vi "运维调试_CODCr.vi"() -> ()   [LabVIEW 2016, in "CODCr库.lvlib"]
uses:
  <vilib>/Utility/miscctls.llb/LVPointTypeDef.ctl
  <vilib>/ptbypt/NI_PtbyPt.lvlib
  <vilib>/Utility/config.llb/NI_LVConfig.lvlib
panel:
  in  "手动模式":bool
  in  "维护模式":bool
  out "数据时间":timestamp format="%<%Y/%m/%d %H:%M:%S>T"
  in  "质控参数":bool
  in  "仪器参数":bool
  in  "MB通信方式选择":enum16{"串口", "TCP"}(ring)
  in  "释放串口":bool
  in  "打开串口":bool
  in  "加标回收测试":bool
  in  "平行样测试":bool
  in  "定时启动":bool
  out "COM口":string
  in  "空白测试":bool
  in  "隐藏按钮":bool
  in  "写入消解温度时长":bool
  in  "保存KB值":bool
  in  "标样核查":bool
  out "启动时间":timestamp format="%<%Y/%m/%d %H:%M:%S>T"
  out "主循环次数":i32
  out "status":bool
  out "启动测量模式":T1(ring)
  out "曲线截距B":sgl format="%#_10g"
  out "曲线斜率K":sgl format="%#_10g"
  out "量程上限":sgl
  out "量程下限":sgl
  out "消解时长":u16
  out "消解温度":u16
  out "测量精度":u16
  out "测量结果":sgl
  out "标样参考值":sgl
  out "量程":u16
  out "工作状态":T1(ring)
  out "仪器时间":timestamp format="%<%X\n%x>T"
  out "关键参数区":T2
  out "状态告警区":T3 {"告警代码" items=["无告警", "缺试剂告警", "缺水样告警", "缺蒸馏水告警", "缺标液告警", "仪表漏液告警", "标定异常告警", "超量程告警", "加热异常", "低试剂预警", "超上限告警", "超下限告警", "仪表内部其他异常", "滴定异常告警", "电极异常告警", "量程切换告警", "参数设置告警", "PH电极电位异常", "电导率电极异常", "浊度光度异常", "溶解氧电极异常", "溶解氧光强异常", "温度异常告警", "PH异常告警", "溶解氧异常告警", "电导率异常告警", "浊度异常告警", "叶绿素异常告警", "藻密度异常告警", "蓝绿藻异常告警", "ORP异常告警", "氨氮异常告警", "清洁刷异常告警", "SD卡异常告警", "蓝牙异常告警", "Wifi异常告警", "流程异常告警"]; "故障代码" items=["无故障", "电机故障", "温度故障", "通讯故障", "滴定故障"]}
  out "测量数据区":T4 {"单位" items=["ug/L", "mg/L", "ppm", "mg/m3", "cm", "ppb", "ug/m3", "%", "nmol/mol", "umol/mol", "MPN/L", "MPN/100ml", "ng/m3", "NTU", "无量纲", "ms/cm", "us/cm", "℃", "mV", "万个/L"]}
  out "系统时间":timestamp format="%<%Y/%m/%d %H:%M:%S>T"
  in  "停止":bool
  in  "校时":bool
  in  "标样校准":bool
  in  "空白校准":bool
  in  "零点核查":bool
  in  "跨度核查":bool
  in  "水样测试":bool
  in  "返回":bool
  in  "设置":bool
  # "mg/L"
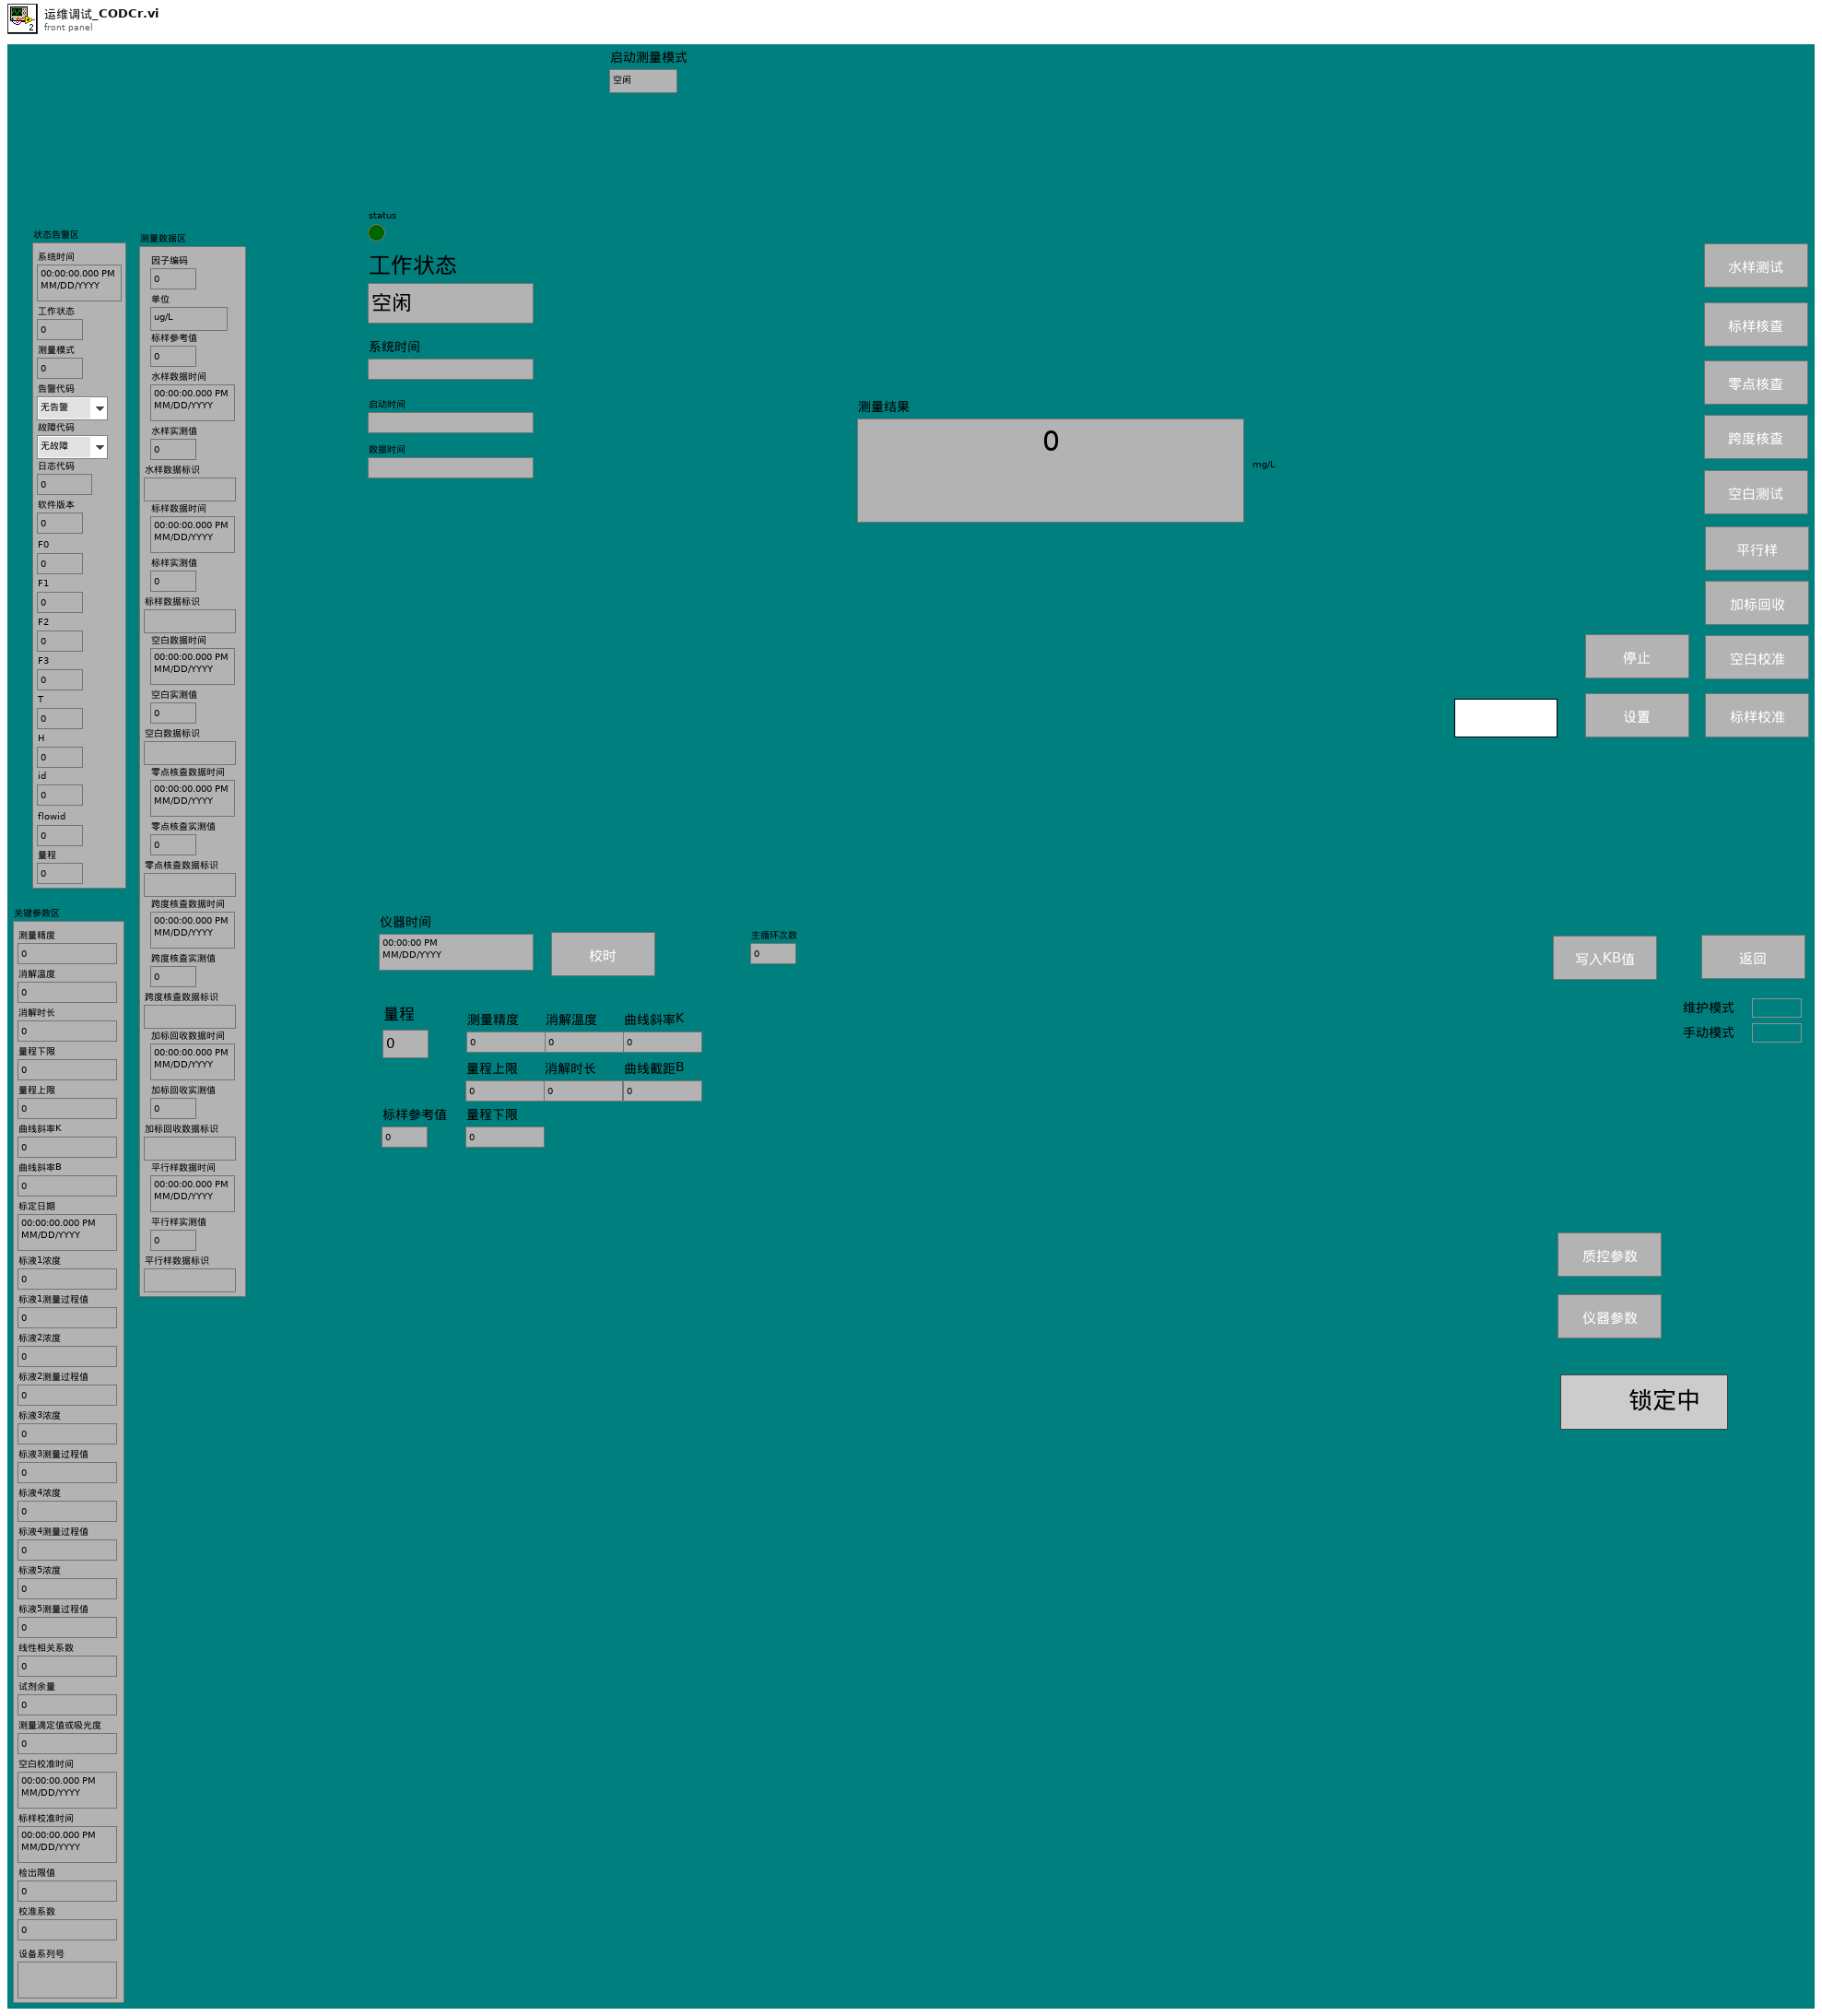
[diagram p1: front panel]
types:
  T1 = enum16{"空闲", "水样测试", "标样核查", "零点核查", "跨度核查", "空白测试", "平行样测试", "加标回收", "空白校准", "标样校准", "初始化（清洗）"}
  T2 = cluster{"测量精度":u16, "消解温度":u16, "消解时长":u16, "量程下限":sgl, "量程上限":sgl, "曲线斜率K":sgl, "曲线斜率B":sgl, "标定日期":timestamp, "标液1浓度":sgl, "标液1测量过程值":sgl, "标液2浓度":sgl, "标液2测量过程值":sgl, "标液3浓度":sgl, "标液3测量过程值":sgl, "标液4浓度":sgl, "标液4测量过程值":sgl, "标液5浓度":sgl, "标液5测量过程值":sgl, "线性相关系数":sgl, "试剂余量":u32, "测量滴定值或吸光度":sgl, "空白校准时间":timestamp, "标样校准时间":timestamp, "检出限值":sgl, "校准系数":sgl, "设备系列号":string}
  T3 = cluster{"系统时间":timestamp, "工作状态":u16, "测量模式":u16, "告警代码":u16, "故障代码":u16, "日志代码":u16, "软件版本":u16, "F0":sgl, "F1":sgl, "F2":sgl, "F3":sgl, "T":sgl, "H":sgl, "id":u16, "flowid":u16, "量程":u16}
  T4 = cluster{"因子编码":u32, "单位":u16, "标样参考值":sgl, "水样数据时间":timestamp, "水样实测值":sgl, "水样数据标识":string, "标样数据时间":timestamp, "标样实测值":sgl, "标样数据标识":string, "空白数据时间":timestamp, "空白实测值":sgl, "空白数据标识":string, "零点核查数据时间":timestamp, "零点核查实测值":sgl, "零点核查数据标识":string, "跨度核查数据时间":timestamp, "跨度核查实测值":sgl, "跨度核查数据标识":string, "加标回收数据时间":timestamp, "加标回收实测值":sgl, "加标回收数据标识":string, "平行样数据时间":timestamp, "平行样实测值":sgl, "平行样数据标识":string}
  T5 = cluster{"命令":string, "测量模式":enum16{"水样测量", "标样核查", "零点核查", "跨度核查", "空白测试", "加标回收", "平行样", "校零", "校标"}, "CODCr量程切换":enum32{"H", "L", "AUTO"}}
  T6 = typedef "LVPointTypeDef.ctl" = cluster{"Horizontal":i16, "Vertical":i16}
  T7 = typedef "NI_LVConfig.lvlib/Config Data RefNum.ctl" = refnum<k1>
  T8 = typedef "报警信息字段定义.ctl" = cluster{"时间":timestamp, "参数":string, "元器件":string, "故障现象":string, "故障分析":string, "state":string, "code":string, "platform_alarm_code":string}
  T9 = cluster{"时间标识":timestamp, "参数":string, "日志信息":string, "流程参数":string}
  T10 = cluster{"测量模式":enum16{"水样测量", "标样核查", "零点核查", "跨度核查", "空白测试", "加标回收", "平行样", "校零", "校标"}}
  T11 = typedef "TimingControl.lvlib/TimingControl.lvclass/国标控制命令.ctl" = enum16{"启动测量", "标样核查", "零点核查", "跨度核查", "空白测试", "平行样测试", "加标回收", "空白校准", "标样校准", "初始化（清洗）", "停止测试", "仪器重启", "校时", "模式设置", "测量间隔设置"}
  T12 = typedef "TimingControl.lvlib/TimingControl.lvclass/测量参数.ctl" = u16
  T13 = cluster{"测量量程":dbl, "测量精度":dbl, "测量间隔":dbl, "消解温度":dbl, "消解时长":dbl, "空白校准时间":timestamp, "曲线截距":dbl, "曲线斜率":dbl, "测量检出限":dbl, "测量信号值":dbl, "线性相关系数":dbl, "二次多项式系数":dbl, "标样校准时间":timestamp, "稀释倍数":dbl, "三项式系数":dbl, "空白标定系数":dbl, "量程系数":dbl}
  T14 = cluster{"确定":bool, "测量量程":dbl, "测量精度":dbl, "测量间隔":dbl, "消解温度":dbl, "消解时长":dbl, "空白校准时间":timestamp, "曲线截距":dbl, "曲线斜率":dbl, "测量检出限":dbl, "测量信号值":dbl, "线性相关系数":dbl, "二次多项式系数":dbl, "标样校准时间":timestamp, "稀释倍数":dbl, "三项式系数":dbl, "空白标定系数":dbl, "量程系数":dbl}
  T15 = cluster{"跨度值":dbl, "零点标准液浓度":dbl, "跨度标准液浓度":dbl, "标准液标准浓度":dbl}
  T16 = cluster{"确定":bool, "跨度值":dbl, "零点标准液浓度":dbl, "跨度标准液浓度":dbl, "标准液标准浓度":dbl}
  T17 = enum16{"水样测量", "标样核查", "零点核查", "跨度核查", "空白测试", "加标回收", "平行样", "校零", "校标"}
  T18 = typedef "CODCr库.lvlib/测试模式.ctl" = enum16{"N", "M"}
  T19 = cluster{"运行模式":enum16{"维护模式", "常规模式", "应急模式", "质控模式"}}
  T20 = cluster{"时间标识":timestamp, "监测值":sgl, "单位":u16, "数据标识":string, "因子编码":u32, "标样参考值":sgl, "F0":sgl, "F1":sgl, "F2":sgl, "F3":sgl, "温度":sgl, "湿度":sgl, "量程标识":string, "LastTime":timestamp}
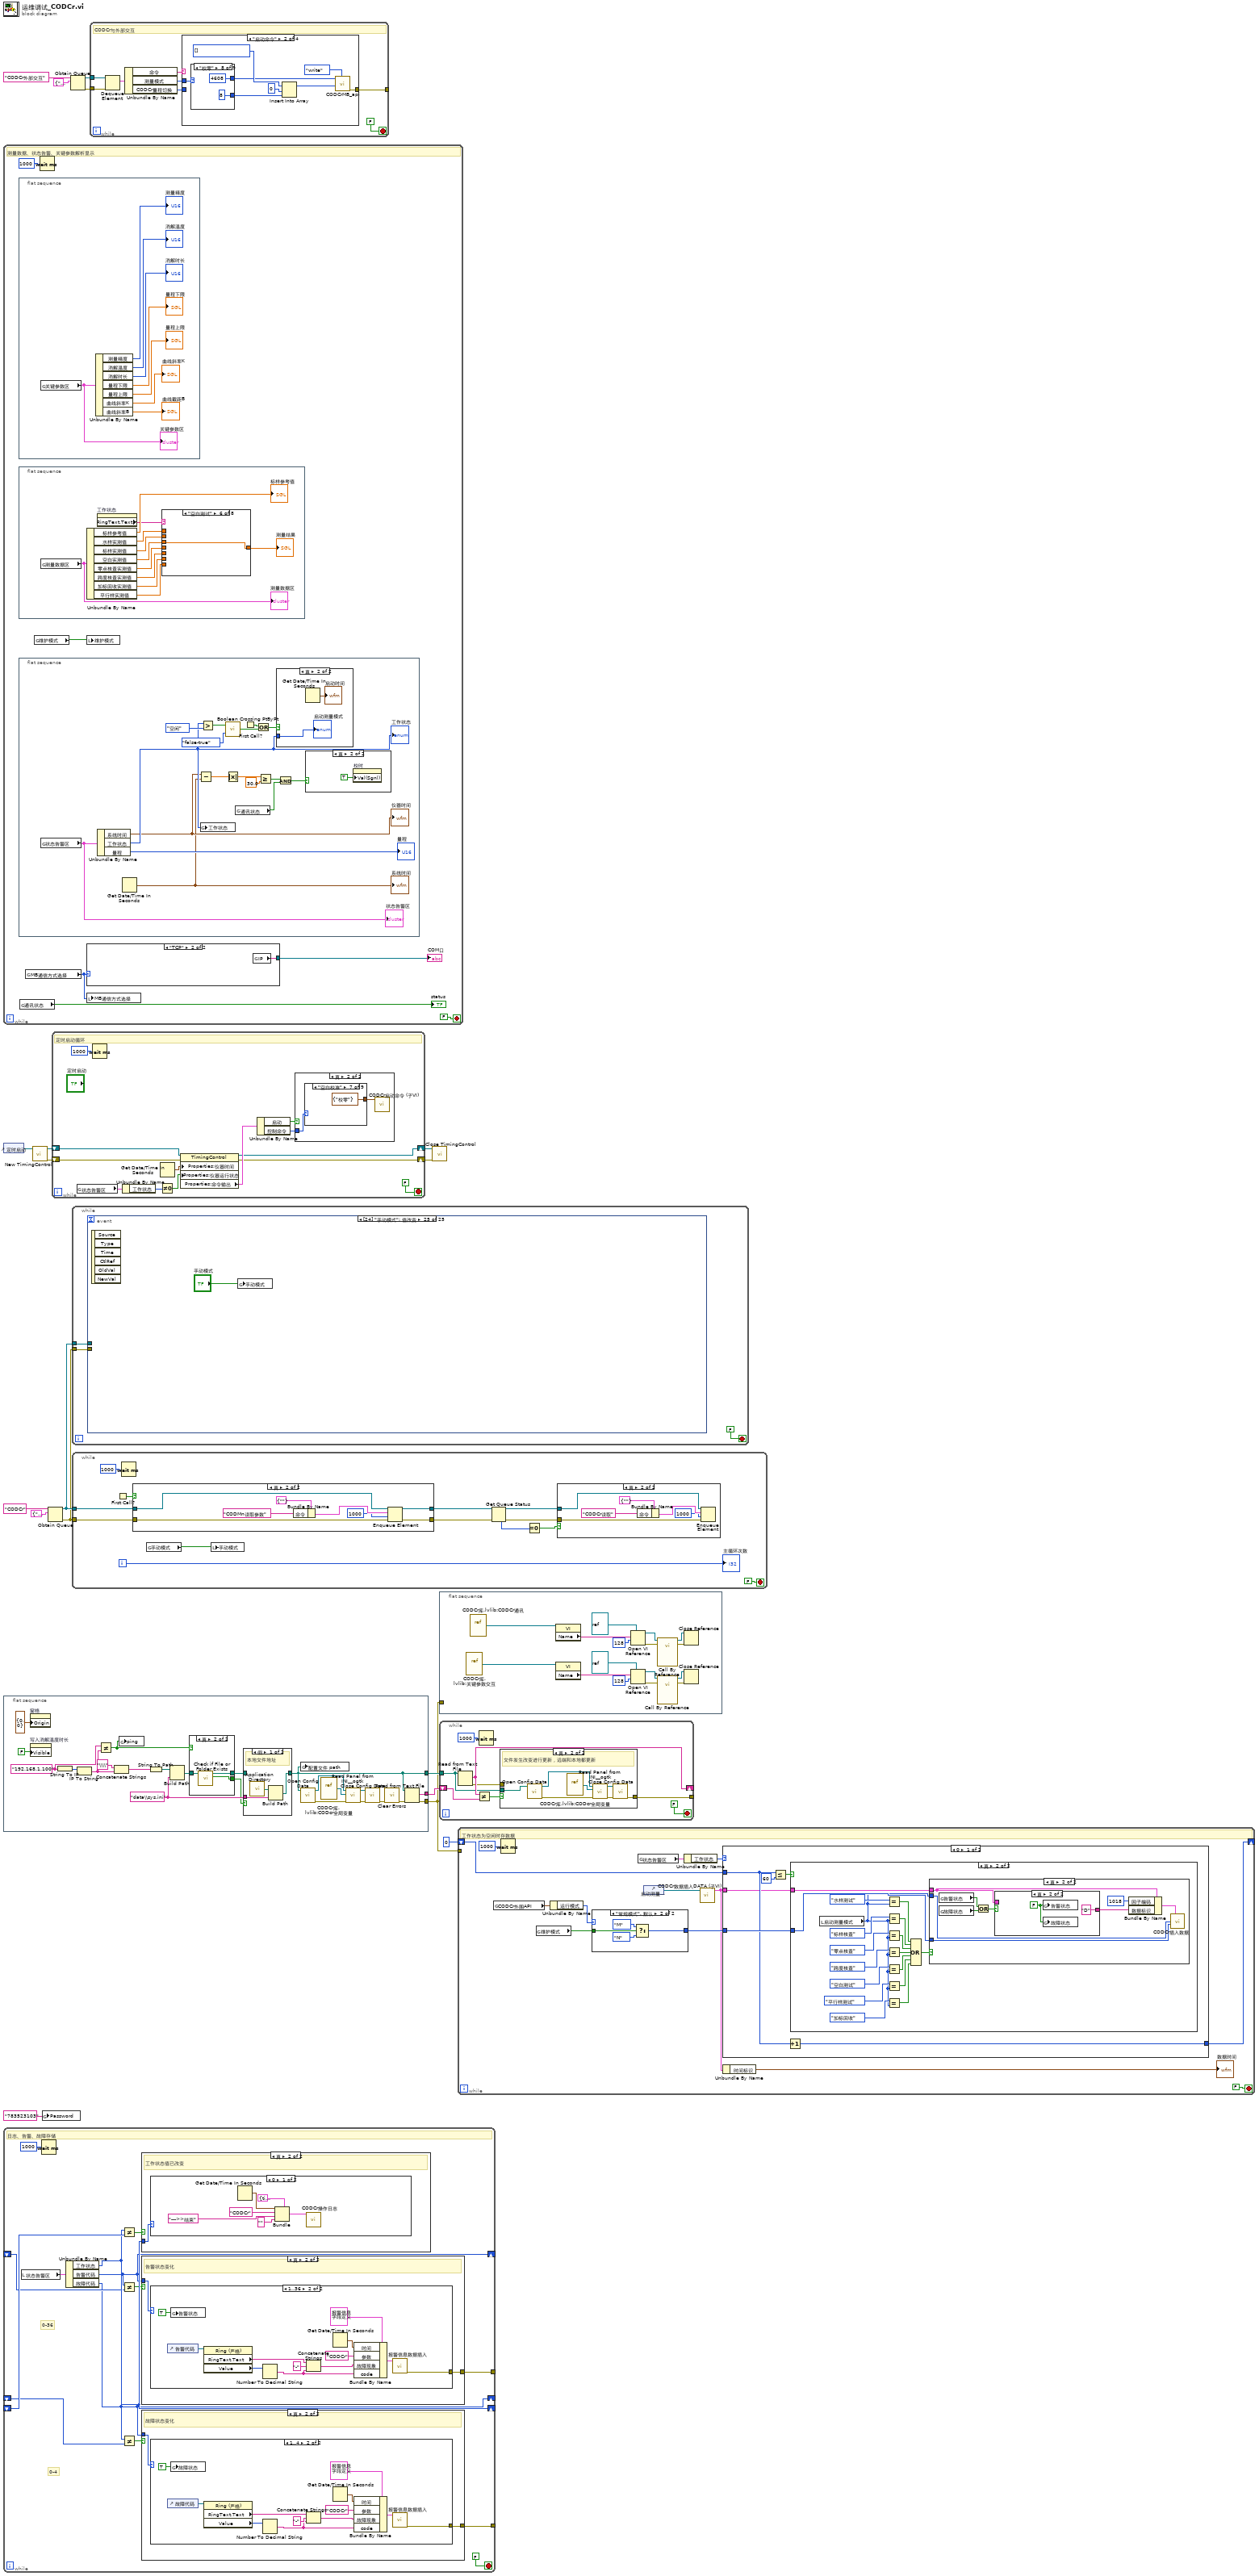
[diagram p0: block diagram]
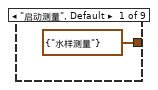
[diagram p3: hidden frame]
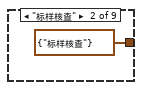
[diagram p4: hidden frame]
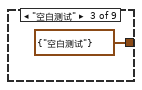
[diagram p5: hidden frame]
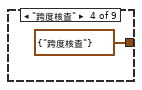
[diagram p6: hidden frame]
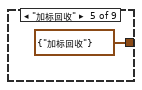
[diagram p7: hidden frame]
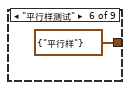
[diagram p8: hidden frame]
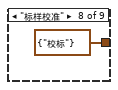
[diagram p9: hidden frame]
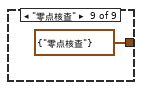
[diagram p10: hidden frame]
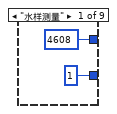
[diagram p15: hidden frame]
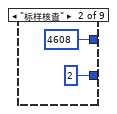
[diagram p16: hidden frame]
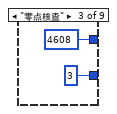
[diagram p17: hidden frame]
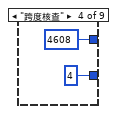
[diagram p18: hidden frame]
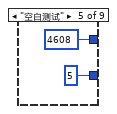
[diagram p19: hidden frame]
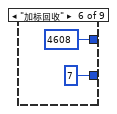
[diagram p20: hidden frame]
diagram:
  n1 = while {
    stop <- FALSE stop-if-true
    # "测量数据、状态告警、关键参数解析显示"
    n2 = flat-sequence {
      frame #0 {
        n3 = global read "CODcr全局变量.vi" "关键参数区"() -> (w27:T2)
        "关键参数区" <- w27
        n4 = Unbundle By Name(w27) -> ("测量精度"=→"测量精度":u16, "消解温度"=→"消解温度":u16, "消解时长"=→"消解时长":u16, "量程下限"=→"量程下限":sgl, "量程上限"=→"量程上限":sgl, "曲线斜率K"=→"曲线斜率K":sgl, "曲线斜率B"=→"曲线截距B":sgl)
      }
    }
    n5 = flat-sequence {
      frame #0 {
        n6 = global read "CODcr全局变量.vi" "测量数据区"() -> (w55:T4)
        "测量数据区" <- w55
        n7 = Unbundle By Name(w55) -> ("标样参考值"=→"标样参考值":sgl, "水样实测值"=w63:sgl, "标样实测值"=w61:sgl, "空白实测值"=w58:sgl, "零点核查实测值"=w60:sgl, "跨度核查实测值"=w59:sgl, "加标回收实测值"=w56:sgl, "平行样实测值"=w57:sgl)
        n8 = property on="工作状态" class="Enum (严格)"() -> ("RingText.Text"=w64:string)  [unwired: 2 in, 2 out]
        n9 = case shown="\"空白测试\"" w64 {
          tunnel: w63 -> [_ w67 _ _ _ _ _ _]
          tunnel: [w66 w67 w68 w69 w70 w71 w72 w73] -> w62
          tunnel: w61 -> [_ _ w68 _ _ _ _ _]
          tunnel: w60 -> [_ _ _ w69 _ _ _ _]
          tunnel: w59 -> [_ _ _ _ w70 _ _ _]
          tunnel: w58 -> [_ _ _ _ _ w71 _ _]
          tunnel: w57 -> [_ _ _ _ _ _ w72 _]
          tunnel: w56 -> [_ _ _ _ _ _ _ w73]
          frame "空闲", Default {
            n10 = local read "测量结果"() -> (w66:sgl)
          }
          frame "水样测试" {
          }
          frame "标样核查" {
          }
          frame "零点核查" {
          }
          frame "跨度核查" {
          }
          frame "空白测试" {
          }
          frame "平行样测试" {
          }
          frame "加标回收" {
          }
        }
        "测量结果" <- w62
      }
    }
    n11 = flat-sequence {
      frame #0 {
        n12 = global read "CODcr全局变量.vi" "状态告警区"() -> (w43:T3)
        "状态告警区" <- w43
        n13 = Unbundle By Name(w43) -> ("系统时间"=w42:timestamp, "工作状态"=w46:u16, "量程"=→"量程":u16)
        "仪器时间" <- w42
        "工作状态" <- w46
        n14 = Get Date/Time In Seconds() -> (seconds since 1Jan1904=w41:timestamp)
        "系统时间" <- w41
        n15 = Subtract(x=w42, y=w41) -> (x-y=w40:dbl)
        n16 = global write "CODcr全局变量.vi" "工作状态"(w46) -> ()
        n17 = Greater?(x=w46, y=T1."空闲") -> (0:w50:bool)
        n18 = call <vilib>:"Boolean Crossing PtByPt.vi"("direction"=enum16{"either", "false-true", "true-false"}."false-true", "input"=w50) -> ("crossing"=w49:bool)  [unwired: 1 in]
        n19 = Absolute Value(x=w40) -> (abs(x)=w39:dbl)
        n20 = global read "CODcr全局变量.vi" "通讯状态"() -> (w35:bool)
        n21 = First Call?() -> (First Call?: T/F=w44:bool)
        n22 = Or(x=w44, y=w49) -> (x .or. y?=w45:bool)
        n23 = Greater Or Equal?(x=w39, y=30.0) -> (x >= y?=w36:bool)
        n24 = case shown="真" w45 {
          tunnel: w46 -> [_ w53]
          frame False {
          }
          frame True {
            n25 = Get Date/Time In Seconds() -> (seconds since 1Jan1904=→"启动时间":timestamp)
            "启动测量模式" <- w53
          }
        }
        n26 = And(x=w36, y=w35) -> (x .and. y?=w37:bool)
        n27 = case shown="真" w37 {
          frame False {
          }
          frame True {
            n28 = property on="校时" class="Bool (严格)"("Val(Sgnl)"=TRUE ("值(信号)")) -> ()  [unwired: 2 in, 2 out]
          }
        }
      }
    }
    n29 = global read "CODcr全局变量.vi" "通讯状态"() -> (→"status":bool)
    n30 = global read "CODcr全局变量.vi" "MB通信方式选择"() -> (w20:enum16{"串口", "TCP"})
    n31 = global read "CODcr全局变量.vi" "维护模式"() -> (w19:bool)
    n32 = Wait (ms)(milliseconds to wait=u32 1000 ("等待时间（毫秒）")) -> ()  [unwired: 1 out]
    n33 = local write "维护模式"(w19) -> ()
    n34 = case shown="\"TCP\"" w20 {
      tunnel: [w25 w26] -> w21
      frame "串口", Default {
        n35 = global read "CODcr全局变量.vi" "VISA Resource"() -> (w25:refnum<visa-resource-name>)
      }
      frame "TCP" {
        n36 = global read "CODcr全局变量.vi" "IP"() -> (w26:string)
      }
    }
    "COM口" <- w21
    n37 = local write "MB通信方式选择"(w20) -> ()
  }
  n38 = control-ref of="定时启动"() -> (w6:refnum<vi>)
  n39 = flat-sequence {
    tunnel: [w76] -> w7
    tunnel: [w75] -> w9
    tunnel: [w74] -> w8
    frame #0 {
      w94 = "data\\sys.ini" ("名称或相对路径")
      w79 = "192.168.1.100" ("名称")
      n40 = property on="窗格" class="Pane"("Origin"=T6 {"Horizontal"=0, "Vertical"=0} ("原点")) -> ()  [unwired: 2 in, 2 out]
      n41 = property on="写入消解温度时长" class="Bool"("Visible"=FALSE ("可见")) -> ()  [unwired: 2 in, 2 out]
      n42 = String To IP(1:w79) -> (0:w86:u32)
      n43 = IP To String(2:w86) -> (0:w83:string)  [unwired: 1 in]
      n44 = Not Equal?(x=w79, y=w83) -> (x != y?=w93:bool)
      n45 = Concatenate Strings("\\\\" ("字符串"), w83) -> (w84:string)
      n46 = global write "CODcr全局变量.vi" "ping"(w93) -> ()
      n47 = String To Path(string=w84) -> (path=w78:path)
      n48 = Build Path(base path=w78, name or relative path=w94) -> (appended path=w82:path)
      n49 = case shown="真" w93 {
        tunnel: w82 -> [w97 w101]
        tunnel: [w97 w100] -> w81
        tunnel: [FALSE w99] -> w80
        frame False {
        }
        frame True {
          n50 = call <vilib>:"Check if File or Folder Exists.vi"("path"=w101) -> ("file or folder exists?"=w99:bool, "dup path"=w100:path)  [unwired: 8 in, 1 out]
        }
      }
      n51 = case shown="假" w80 {
        tunnel: w81 -> [_ w105]
        tunnel: [w103 w105] -> w74
        tunnel: w94 -> [w102 _]
        frame False {
          # "本地文件地址"
          n52 = call <vilib>:"Application Directory.vi"() -> ("Application Directory"=w104:path)
          n53 = Build Path(base path=w104, name or relative path=w102) -> (appended path=w103:path)
        }
        frame True {
          # "网络共享地址"
        }
      }
      n54 = global write "CODcr全局变量.vi" "配置文件 path"(w74) -> ()
      n55 = call <vilib>:"Open Config Data.vi"("configuration file path"=w74) -> ("error out"=w90:errorcluster, "refnum"=w89:T7)  [unwired: 8 in, 1 out]
      n56 = vi-ref "CODCr库.lvlib:CODcr全局变量.vi"() -> (w77:refnum<vi>)
      n57 = call <userlib>:"Read Panel from INI__ogtk.vi"("error in (no error)"=w90, "VI ref"=w77, "refnum"=w89) -> ("error out"=w88:errorcluster, "refnum out"=w87:T7)  [unwired: 7 in]
      n58 = call <vilib>:"Close Config Data.vi"("error in (no error)"=w88, "refnum"=w87) -> ("error out"=w91:errorcluster)  [unwired: 8 in, 1 out]
      n59 = call <vilib>:"Clear Errors.vi"("error in (no error)"=w91) -> ("error out"=w92:errorcluster)  [unwired: 5 in, 1 out]
      n60 = Read from Text File(file (use dialog)=w74, error in=w92) -> (text=w75:string, error out=w76:errorcluster)  [unwired: 2 in, 2 out]
    }
  }
  n61 = while {
    shift-right: [w115] -> _
    shift-left: _ -> [w117]
    shift-right: [w112] -> _
    shift-left: _ -> [w113]
    shift-right: [w108] -> _
    shift-left: _ -> [w110]
    tunnel: [w109] -> _
    tunnel: [w107] -> _
    stop <- FALSE stop-if-true
    # "0-4"
    # "0-36"
    # "日志、告警、故障存储"
    n62 = local read "状态告警区"() -> (w106:T3)
    n63 = Wait (ms)(milliseconds to wait=u32 1000 ("等待时间（毫秒）")) -> ()  [unwired: 1 out]
    n64 = Unbundle By Name(w106) -> ("工作状态"=w115:u16, "告警代码"=w112:u16, "故障代码"=w108:u16)
    n65 = Not Equal?(x=w115, y=w117) -> (x != y?=w116:bool)
    n66 = Not Equal?(x=w112, y=w113) -> (x != y?=w114:bool)
    n67 = Not Equal?(x=w108, y=w110) -> (x != y?=w111:bool)
    n68 = case shown="真" w116 {
      tunnel: w115 -> [_ w148]
      frame False {
      }
      frame True {
        # "工作状态值已改变"
        n69 = case shown="0" w148 {
          frame 0 {
            n70 = Get Date/Time In Seconds() -> (seconds since 1Jan1904=w150:timestamp)
            n71 = Bundle(cluster=T9 {"时间标识"=timestamp(0 s since 1904-01-01), "参数"="", "日志信息"="", "流程参数"=""} ("data in"), "时间标识"=w150, "参数"="CODCr" ("table输入"), "日志信息"="--->>结束", "流程参数"="" ("table输入")) -> (w149:T9)
            n72 = call "CODCr操作日志.vi"("data"=w149) -> ()  [unwired: 11 in]
          }
          frame 1, Default {
            n73 = property on="工作状态" class="Enum (严格)"() -> ("RingText.Text"=w156:string)  [unwired: 2 in, 2 out]
            n74 = Concatenate Strings("--->>启动" ("日志信息"), w156) -> (w157:string)
            n75 = Get Date/Time In Seconds() -> (seconds since 1Jan1904=w159:timestamp)
            n76 = Bundle(cluster=T9 {"时间标识"=timestamp(0 s since 1904-01-01), "参数"="", "日志信息"="", "流程参数"=""} ("data in"), "时间标识"=w159, "参数"="CODCr" ("table输入"), "日志信息"=w157, "流程参数"="" ("table输入")) -> (w155:T9)
            n77 = call "CODCr操作日志.vi"("data"=w155) -> ()  [unwired: 11 in]
          }
        }
      }
    }
    n78 = case shown="真" w114 {
      tunnel: w112 -> [_ w135]
      tunnel: [_ w134] -> w109
      frame False {
      }
      frame True {
        # "告警状态变化"
        n79 = case shown="1..36" w135 {
          tunnel: [_ w139] -> w134
          frame 0, Default {
            # "无告警"
          }
          frame 1..36 {
            n80 = control-ref of="告警代码"() -> (w145:refnum<vi>)
            n81 = global write "CODcr全局变量.vi" "告警状态"(TRUE ("告警状态")) -> ()
            n82 = property class="Ring (严格)"(reference=w145) -> ("RingText.Text"=w143:string, "Value"=w142:u16)  [unwired: 1 in, 2 out]
            n83 = Number To Decimal String(number=w142) -> (decimal integer string=w136:string)  [unwired: 1 in]
            n84 = Concatenate Strings(w143, "-" ("字符串"), w136) -> (w141:string)
            n85 = Get Date/Time In Seconds() -> (seconds since 1Jan1904=w147:timestamp)
            n86 = Bundle By Name(cluster=T8 {"时间"=timestamp(0 s since 1904-01-01), "参数"="水样测试", "元器件"="N", "故障现象"="", "故障分析"="", "state"="", "code"="", "platform_alarm_code"=""} ("data"), "时间"=w147, "参数"="CODCr" ("table输入"), "故障现象"=w141, "code"=w136) -> (w137:T8)
            n87 = call "报警信息数据插入.vi"("data"=w137) -> ("错误输出"=w139:errorcluster)  [unwired: 9 in]
          }
        }
      }
    }
    n88 = case shown="真" w111 {
      tunnel: w108 -> [_ w121]
      tunnel: [_ w120] -> w107
      frame False {
      }
      frame True {
        # "故障状态变化"
        n89 = case shown="1..4" w121 {
          tunnel: [_ w123] -> w120
          frame 0, Default {
            # "无告警"
          }
          frame 1..4 {
            n90 = control-ref of="故障代码"() -> (w133:refnum<vi>)
            n91 = global write "CODcr全局变量.vi" "故障状态"(TRUE ("告警状态")) -> ()
            n92 = property class="Ring (严格)"(reference=w133) -> ("RingText.Text"=w128:string, "Value"=w129:u16)  [unwired: 1 in, 2 out]
            n93 = Number To Decimal String(number=w129) -> (decimal integer string=w122:string)  [unwired: 1 in]
            n94 = Concatenate Strings(w128, "-" ("字符串"), w122) -> (w127:string)
            n95 = Get Date/Time In Seconds() -> (seconds since 1Jan1904=w131:timestamp)
            n96 = Bundle By Name(cluster=T8 {"时间"=timestamp(0 s since 1904-01-01), "参数"="水样测试", "元器件"="N", "故障现象"="", "故障分析"="", "state"="", "code"="", "platform_alarm_code"=""} ("data"), "时间"=w131, "参数"="CODCr" ("table输入"), "故障现象"=w127, "code"=w122) -> (w125:T8)
            n97 = call "报警信息数据插入.vi"("data"=w125) -> ("错误输出"=w123:errorcluster)  [unwired: 9 in]
          }
        }
      }
    }
  }
  n98 = call "New TimingControl.vi"("Reference"=w6) -> ("error out"=w4:errorcluster, "TimingControl out"=w5:refnum<class "TimingControl.lvclass">)  [unwired: 9 in]
  n99 = global write "外部调用接口全局变量.vi" "Password"("783523103" ("Password")) -> ()
  n100 = Obtain Queue(name (unnamed)="CODCr" ("名称（未命名）"), element data type=cluster{"命令":string} {"命令"="启用模块"} ("元素")) -> (queue out=w12:refnum<queue>, error out=w11:errorcluster)  [unwired: 3 in, 1 out]
  n101 = while {
    shift-right: [w167] -> w3
    shift-left: w5 -> [w173]
    shift-right: [w166] -> w2
    shift-left: w4 -> [w172]
    stop <- FALSE stop-if-true
    # "定时启动循环"
    n102 = global read "CODcr全局变量.vi" "状态告警区"() -> (w169:T3)
    n103 = Wait (ms)(milliseconds to wait=u32 1000 ("等待时间（毫秒）")) -> ()  [unwired: 1 out]
    n104 = Unbundle By Name(w169) -> ("工作状态"=w165:u16)
    n105 = Not Equal To 0?(x=w165) -> (x != 0?=w168:bool)
    n106 = Get Date/Time In Seconds() -> (seconds since 1Jan1904=w171:timestamp)
    n107 = property class="TimingControl"(reference=w173, error in=w172, "Properties:仪器时间"=w171, "Properties:仪器运行状态"=w168) -> (reference out=w167:refnum<class "TimingControl.lvclass">, error out=w166:errorcluster, "Properties:命令输出"=w170:cluster{"启动":bool, "控制命令":T11, "测量参数":T12})
    n108 = Unbundle By Name(w170) -> ("启动"=w163:bool, "控制命令"=w164:T11)
    n109 = case shown="真" w163 {
      tunnel: w164 -> [_ w177]
      frame False {
      }
      frame True {
        n110 = case shown="\"空白校准\"" w177 {
          tunnel: [T10 {"测量模式"=enum."水样测量"} ("启动测量模式") T10 {"测量模式"=enum."标样核查"} ("启动测量模式") T10 {"测量模式"=enum."空白测试"} ("启动测量模式") T10 {"测量模式"=enum."跨度核查"} ("启动测量模式") T10 {"测量模式"=enum."加标回收"} ("启动测量模式") T10 {"测量模式"=enum."平行样"} ("启动测量模式") T10 {"测量模式"=enum."校零"} ("启动测量模式") T10 {"测量模式"=enum."校标"} ("启动测量模式") T10 {"测量模式"=enum."零点核查"} ("启动测量模式")] -> w176
          frame "启动测量", Default {
          }
          frame "标样核查" {
          }
          frame "空白测试" {
          }
          frame "跨度核查" {
          }
          frame "加标回收" {
          }
          frame "平行样测试" {
          }
          frame "空白校准" {
          }
          frame "标样校准" {
          }
          frame "零点核查" {
          }
        }
        n111 = call "CODCr启动命令 (子VI).vi"("启动测量模式"=w176) -> ()  [unwired: 11 in]
      }
    }
  }
  n112 = Obtain Queue(name (unnamed)="CODCr外部交互" ("名称（未命名）"), element data type=T5 {"命令"="启动命令", "测量模式"=enum."水样测量", "CODCr量程切换"=enum."AUTO"} ("元素")) -> (queue out=w14:refnum<queue>, error out=w13:errorcluster)  [unwired: 3 in, 1 out]
  n113 = while {
    tunnel: w12 -> [w188]
    tunnel: w11 -> [w187]
    stop <- FALSE stop-if-true
    n114 = event shown="[24] \"手动模式\": 值改变" {
      selector: _ -> [_ _ _ _ _ _ _ _ _ _ _ _ _ _ _ _ _ _ _ _ _ _ _ _ _]
      dyn-events: _ -> [_ _ _ _ _ _ _ _ _ _ _ _ _ _ _ _ _ _ _ _ _ _ _ _ _]
      timeout: _ -> [_ _ _ _ _ _ _ _ _ _ _ _ _ _ _ _ _ _ _ _ _ _ _ _ _]
      tunnel: w188 -> [_ _ _ _ _ _ _ _ _ _ _ _ _ _ _ w287 w306 _ _ _ w330 _ _ _ _]
      tunnel: w187 -> [_ _ _ _ _ _ _ _ _ _ _ _ _ _ _ w286 w305 _ _ _ w329 _ _ _ _]
      event Timeout {
        n115 = event-data() -> ()  [unwired: 1 in, 2 out]
      }
      event "水样测试": Value Change {
        n116 = event-data() -> ()  [unwired: 1 in, 6 out]
        n117 = local write "启动测量模式"(T1."水样测试" ("启动测量模式")) -> ()
        n118 = call "CODCrMB_api.vi"("STEP"=enum16{"open", "read", "write", "close"}."write", "values"=u16[] [1], "starting address"=u16 4608) -> ()  [unwired: 6 in, 3 out]
      }
      event "标样核查": Value Change {
        n119 = event-data() -> ()  [unwired: 1 in, 6 out]
        n120 = local write "启动测量模式"(T1."标样核查" ("启动测量模式")) -> ()
        n121 = call "CODCrMB_api.vi"("STEP"=enum16{"open", "read", "write", "close"}."write", "values"=u16[] [2], "starting address"=u16 4608) -> ()  [unwired: 6 in, 3 out]
      }
      event "零点核查": Value Change {
        n122 = event-data() -> ()  [unwired: 1 in, 6 out]
        n123 = local write "启动测量模式"(T1."零点核查" ("启动测量模式")) -> ()
        n124 = call "CODCrMB_api.vi"("STEP"=enum16{"open", "read", "write", "close"}."write", "values"=u16[] [3], "starting address"=u16 4608) -> ()  [unwired: 6 in, 3 out]
      }
      event "跨度核查": Value Change {
        n125 = event-data() -> ()  [unwired: 1 in, 6 out]
        n126 = local write "启动测量模式"(T1."跨度核查" ("启动测量模式")) -> ()
        n127 = call "CODCrMB_api.vi"("STEP"=enum16{"open", "read", "write", "close"}."write", "values"=u16[] [4], "starting address"=u16 4608) -> ()  [unwired: 6 in, 3 out]
      }
      event "空白测试": Value Change {
        n128 = event-data() -> ()  [unwired: 1 in, 6 out]
        n129 = local write "启动测量模式"(T1."空白测试" ("启动测量模式")) -> ()
        n130 = call "CODCrMB_api.vi"("STEP"=enum16{"open", "read", "write", "close"}."write", "values"=u16[] [5], "starting address"=u16 4608) -> ()  [unwired: 6 in, 3 out]
      }
      event "平行样测试": Value Change {
        n131 = event-data() -> ()  [unwired: 1 in, 6 out]
        n132 = local write "启动测量模式"(T1."平行样测试" ("启动测量模式")) -> ()
        n133 = call "CODCrMB_api.vi"("STEP"=enum16{"open", "read", "write", "close"}."write", "values"=u16[] [6], "starting address"=u16 4608) -> ()  [unwired: 6 in, 3 out]
      }
      event "加标回收测试": Value Change {
        n134 = event-data() -> ()  [unwired: 1 in, 6 out]
        n135 = local write "启动测量模式"(T1."加标回收" ("启动测量模式")) -> ()
        n136 = call "CODCrMB_api.vi"("STEP"=enum16{"open", "read", "write", "close"}."write", "values"=u16[] [7], "starting address"=u16 4608) -> ()  [unwired: 6 in, 3 out]
      }
      event "空白校准": Value Change {
        n137 = event-data() -> ()  [unwired: 1 in, 6 out]
        n138 = local write "启动测量模式"(T1."空白校准" ("启动测量模式")) -> ()
        n139 = call "CODCrMB_api.vi"("STEP"=enum16{"open", "read", "write", "close"}."write", "values"=u16[] [8], "starting address"=u16 4608) -> ()  [unwired: 6 in, 3 out]
      }
      event "标样校准": Value Change {
        n140 = event-data() -> ()  [unwired: 1 in, 6 out]
        n141 = local write "启动测量模式"(T1."标样校准" ("启动测量模式")) -> ()
        n142 = call "CODCrMB_api.vi"("STEP"=enum16{"open", "read", "write", "close"}."write", "values"=u16[] [9], "starting address"=u16 4608) -> ()  [unwired: 6 in, 3 out]
      }
      event "停止": Value Change {
        n143 = event-data() -> ()  [unwired: 1 in, 6 out]
        n144 = Two Button Dialog(message="确认是否停止？" ("消息"), 1:"否" ("F按钮名称（“取消”）"), 2:"是" ("T按钮名称（“确定”）")) -> (T button?=w226:bool)
        n145 = case shown="真" w226 {
          frame False {
          }
          frame True {
            n146 = Obtain Notifier(name (unnamed)="CODCr" ("名称（未命名）"), notification data type=FALSE) -> (notifier out=w234:refnum<notifier>, error out=w232:errorcluster)  [unwired: 2 in, 1 out]
            n147 = Send Notification(notification=TRUE ("通知"), notifier=w234, error in (no error)=w232) -> (notifier out=w231:refnum<notifier>, error out=w230:errorcluster)
            n148 = call "CODCrMB_api.vi"("STEP"=enum16{"open", "read", "write", "close"}."write", "values"=u16[] [12], "starting address"=u16 4608) -> ()  [unwired: 6 in, 3 out]
            n149 = Release Notifier(notifier=w231, error in (no error)=w230) -> ()  [unwired: 1 in, 3 out]
          }
        }
      }
      event "保存KB值": Value Change {
        n150 = event-data() -> ()  [unwired: 1 in, 6 out]
        n151 = local read "曲线截距B"() -> (w240:sgl)
        n152 = local read "曲线斜率K"() -> (w241:sgl)
        n153 = Build Array(w241, w240) -> (w246:sgl[])
        n154 = call "FloatToHex.vi"("浮点数"=w246) -> ("DCBA整形输出"=w243:u16[])  [unwired: 10 in]
        n155 = call "CODCrMB_api.vi"("STEP"=enum16{"open", "read", "write", "close"}."write", "values"=w243, "starting address"=u16 4263) -> ("error out"=w242:errorcluster)  [unwired: 6 in, 2 out]
        n156 = case shown="无错误" w242 {
          tunnel: w241 -> [w248 _]
          tunnel: w240 -> [w247 _]
          frame No Error {
            n157 = global read "CODcr全局变量.vi" "CODCr仪器参数"() -> (w250:T13)
            n158 = Bundle By Name(cluster=w250, "曲线截距"=w247, "曲线斜率"=w248) -> (w249:T13)
            n159 = global write "CODcr全局变量.vi" "CODCr仪器参数"(w249) -> ()
          }
          frame Error {
          }
        }
      }
      event "仪器参数": Value Change {
        n160 = event-data() -> ()  [unwired: 1 in, 6 out]
        n161 = global read "CODcr全局变量.vi" "CODCr仪器参数"() -> (w251:T13)
        n162 = call "仪器参数设置.vi"("codcr仪器参数"=w251) -> ("仪器参数设置输出"=w252:T14)  [unwired: 10 in]
        n163 = Unbundle By Name(w252) -> ("确定"=w253:bool)
        n164 = case shown="真" w253 {
          tunnel: w252 -> [_ w255]
          tunnel: w251 -> [_ w254]
          frame False {
          }
          frame True {
            n165 = flat-sequence {
              tunnel: w255 -> [w258]
              tunnel: w254 -> [w256]
              frame #0 {
                n166 = Unbundle By Name(w258) -> ("测量量程"=w272:dbl, "测量精度"=w271:dbl, "测量间隔"=w270:dbl, "消解温度"=w269:dbl, "消解时长"=w268:dbl, "空白校准时间"=w267:timestamp, "曲线截距"=w266:dbl, "曲线斜率"=w265:dbl, "测量检出限"=w264:dbl, "测量信号值"=w263:dbl, "线性相关系数"=w262:dbl, "二次多项式系数"=w261:dbl, "标样校准时间"=w260:timestamp, "稀释倍数"=w259:dbl)
                n167 = Bundle By Name(cluster=w256, "测量量程"=w272, "测量精度"=w271, "测量间隔"=w270, "消解温度"=w269, "消解时长"=w268, "空白校准时间"=w267, "曲线截距"=w266, "曲线斜率"=w265, "测量检出限"=w264, "测量信号值"=w263, "线性相关系数"=w262, "二次多项式系数"=w261, "标样校准时间"=w260, "稀释倍数"=w259) -> (w257:T13)
                n168 = global write "CODcr全局变量.vi" "CODCr仪器参数"(w257) -> ()
              }
              frame #1 {
                n169 = call "配置文件保存.vi"() -> ()  [unwired: 12 in]
              }
            }
          }
        }
      }
      event "维护模式": Value Change {
        n170 = event-data() -> ()  [unwired: 1 in, 6 out]
        n171 = flat-sequence {
          frame #0 {
            n172 = global write "CODcr全局变量.vi" "维护模式"("维护模式") -> ()
          }
          frame #1 {
            n173 = call "配置文件保存.vi"() -> ()  [unwired: 12 in]
          }
        }
      }
      event "质控参数": Value Change {
        n174 = event-data() -> ()  [unwired: 1 in, 6 out]
        n175 = global read "CODcr全局变量.vi" "质控参数设置"() -> (w275:T15)
        n176 = call "质控参数设置.vi"("质控参数设置"=w275) -> ("输出簇"=w274:T16)  [unwired: 10 in]
        n177 = Unbundle By Name(w274) -> ("确定"=w276:bool)
        n178 = case shown="真" w276 {
          tunnel: w275 -> [_ w278]
          tunnel: w274 -> [_ w277]
          frame False {
          }
          frame True {
            n179 = flat-sequence {
              tunnel: w278 -> [w285]
              tunnel: w277 -> [w284]
              frame #0 {
                n180 = Unbundle By Name(w284) -> ("跨度值"=w282:dbl, "零点标准液浓度"=w281:dbl, "跨度标准液浓度"=w280:dbl, "标准液标准浓度"=w279:dbl)
                n181 = Bundle By Name(cluster=w285, "跨度值"=w282, "零点标准液浓度"=w281, "跨度标准液浓度"=w280, "标准液标准浓度"=w279) -> (w283:T15)
                n182 = global write "CODcr全局变量.vi" "质控参数设置"(w283) -> ()
              }
              frame #1 {
                n183 = call "配置文件保存.vi"() -> ()  [unwired: 12 in]
              }
            }
          }
        }
      }
      event "打开串口": Value Change {
        n184 = event-data() -> ()  [unwired: 1 in, 6 out]
        n185 = flat-sequence {
          tunnel: w287 -> [w289]
          tunnel: w286 -> [w288]
          frame #0 {
            n186 = global read "CODcr全局变量.vi" "VISA Resource"() -> (w296:refnum<visa-resource-name>)
            n187 = global read "CODcr全局变量.vi" "PORT"() -> (w290:string)
            n188 = global read "CODcr全局变量.vi" "IP"() -> (w291:string)
            n189 = call "串口配置.vi"("PORT"=w290, "IP"=w291, "请选择串口:"=w296) -> ("PORT 2"=w292:string, "IP 2"=w293:string, "确认 2"=w295:bool, "VISA资源名称 2"=w294:refnum<visa-resource-name>)  [unwired: 5 in]
            n190 = case shown="真" w295 {
              tunnel: w294 -> [_ w299]
              tunnel: w289 -> [_ w301]
              tunnel: w288 -> [_ w300]
              tunnel: w293 -> [_ w298]
              tunnel: w292 -> [_ w297]
              frame False {
              }
              frame True {
                n191 = global write "CODcr全局变量.vi" "IP"(w298) -> ()
                n192 = global write "CODcr全局变量.vi" "PORT"(w297) -> ()
                n193 = global write "CODcr全局变量.vi" "VISA Resource"(w299) -> ()
                n194 = Bundle By Name(cluster=cluster{"命令":string} {"命令"=""} ("元素"), "命令"="启用模块" ("名称（未命名）")) -> (w302:cluster{"命令":string})
                n195 = Enqueue Element(queue=w301, element=w302, error in (no error)=w300) -> ()  [unwired: 1 in, 3 out]
              }
            }
          }
          frame #1 {
            n196 = call "配置文件保存.vi"() -> ()  [unwired: 12 in]
          }
        }
      }
      event "释放串口": Value Change {
        n197 = event-data() -> ()  [unwired: 1 in, 6 out]
        n198 = Two Button Dialog(message="确认是否释放串口，释放串口将导致通信失败！" ("消息")) -> (T button?=w307:bool)  [unwired: 2 in]
        n199 = case shown="真" w307 {
          tunnel: w306 -> [_ w310]
          tunnel: w305 -> [_ w309]
          frame False {
          }
          frame True {
            n200 = Bundle By Name(cluster=cluster{"命令":string} {"命令"=""} ("元素"), "命令"="停用模块" ("名称（未命名）")) -> (w311:cluster{"命令":string})
            n201 = Enqueue Element(queue=w310, element=w311, error in (no error)=w309) -> ()  [unwired: 1 in, 3 out]
          }
        }
      }
      event "MB通信方式选择": Value Change {
        n202 = event-data() -> ()  [unwired: 1 in, 6 out]
        n203 = flat-sequence {
          frame #0 {
            n204 = global write "CODcr全局变量.vi" "MB通信方式选择"("MB通信方式选择") -> ()
          }
          frame #1 {
            n205 = call "配置文件保存.vi"() -> ()  [unwired: 12 in]
          }
        }
      }
      event "写入消解温度时长": Value Change {
        n206 = event-data() -> ()  [unwired: 1 in, 6 out]
        n207 = local read "消解温度"() -> (w320:u16)
        n208 = local read "消解时长"() -> (w319:u16)
        n209 = Build Array(w320, w319) -> (w318:u16[])
        n210 = call "WordToHex.vi"("WORD"=w318) -> ("数组"=w315:u16[])  [unwired: 10 in]
        n211 = call "CODCrMB_api.vi"("STEP"=enum16{"open", "read", "write", "close"}."write", "values"=w315, "starting address"=u16 4257) -> ()  [unwired: 6 in, 3 out]
      }
      event "校时": Value Change {
        n212 = event-data() -> ()  [unwired: 1 in, 6 out]
        n213 = Get Date/Time In Seconds() -> (seconds since 1Jan1904=w328:timestamp)
        n214 = Build Array(w328) -> (w325:timestamp[])
        n215 = call "DateToHex.vi"("DATE"=w325) -> ("数组"=w324:u16[])  [unwired: 10 in]
        n216 = Insert Into Array(array=u16[] [13] ("values"), index=1 ("索引"), new element=w324) -> (w321:u16[])
        n217 = call "CODCrMB_api.vi"("STEP"=enum16{"open", "read", "write", "close"}."write", "values"=w321, "starting address"=u16 4608) -> ()  [unwired: 6 in, 3 out]
      }
      event "设置": Value Change {
        n218 = event-data() -> ()  [unwired: 1 in, 6 out]
        n219 = property on="窗格" class="Pane"("Origin"=T6 {"Horizontal"=0, "Vertical"=728} ("原点")) -> ()  [unwired: 2 in, 2 out]
        n220 = Bundle By Name(cluster=cluster{"命令":string} {"命令"=""} ("元素"), "命令"="CODCr读取参数" ("名称（未命名）")) -> (w331:cluster{"命令":string})
        n221 = Enqueue Element(queue=w330, element=w331, error in (no error)=w329) -> ()  [unwired: 1 in, 3 out]
      }
      event "返回": Value Change {
        w335 = FALSE ("可见")
        n222 = event-data() -> ()  [unwired: 1 in, 6 out]
        n223 = property on="窗格" class="Pane"("Origin"=T6 {"Horizontal"=0, "Vertical"=0} ("原点")) -> ()  [unwired: 2 in, 2 out]
        n224 = property on="打开串口" class="Bool"("Visible"=w335) -> ()  [unwired: 2 in, 2 out]
        n225 = property on="释放串口" class="Bool"("Visible"=w335) -> ()  [unwired: 2 in, 2 out]
        n226 = property on="MB通信方式选择" class="Enum (严格)"("Visible"=w335) -> ()  [unwired: 2 in, 2 out]
        n227 = property on="写入消解温度时长" class="Bool"("Visible"=w335) -> ()  [unwired: 2 in, 2 out]
      }
      event "曲线斜率K", "曲线截距B", "消解温度", "消解时长": Mouse Down {
        n228 = event-data() -> ("CtlRef"=w339:refnum<vi>)  [unwired: 1 in, 7 out]
        n229 = property class="DigNum"(reference=w339) -> (reference out=w340:refnum<vi>, "Value"=w338:variant)  [unwired: 1 in, 1 out]
        n230 = Variant To Data(Variant=w338) -> (data=w337:sgl)  [unwired: 2 in, 1 out]
        n231 = call "CODCR数字键盘.vi"("OldNumber"=w337) -> ("NewNumber"=w341:sgl)
        n232 = property class="DigNum"(reference=w340, "Value"=w341) -> ()  [unwired: 1 in, 2 out]
      }
      event "隐藏按钮": Value Change {
        n233 = event-data() -> ("NewVal"=w342:bool)  [unwired: 1 in, 5 out]
        n234 = property on="打开串口" class="Bool"("Visible"=w342) -> ()  [unwired: 2 in, 2 out]
        n235 = property on="释放串口" class="Bool"("Visible"=w342) -> ()  [unwired: 2 in, 2 out]
        n236 = property on="MB通信方式选择" class="Enum (严格)"("Visible"=w342) -> ()  [unwired: 2 in, 2 out]
        n237 = property on="写入消解温度时长" class="Bool"("Visible"=w342) -> ()  [unwired: 2 in, 2 out]
      }
      event "手动模式": Value Change {
        n238 = event-data() -> ()  [unwired: 1 in, 6 out]
        n239 = global write "CODCr外部API.vi" "手动模式"("手动模式") -> ()
      }
    }
  }
  n240 = while {
    tunnel: w12 -> [w346]
    tunnel: w11 -> [w345]
    i -> [w354]
    stop <- FALSE stop-if-true
    n241 = First Call?() -> (First Call?: T/F=w349:bool)
    n242 = Wait (ms)(milliseconds to wait=u32 1000 ("等待时间（毫秒）")) -> ()  [unwired: 1 out]
    n243 = case shown="真" w349 {
      tunnel: w346 -> [w358 w363]
      tunnel: w345 -> [w357 w362]
      tunnel: [w358 w361] -> w348
      tunnel: [w357 w360] -> w347
      frame False {
      }
      frame True {
        n244 = Bundle By Name(cluster=cluster{"命令":string} {"命令"=""} ("元素"), "命令"="CODMn读取参数" ("名称（未命名）")) -> (w366:cluster{"命令":string})
        n245 = Enqueue Element(queue=w363, element=w366, timeout in ms (-1)=1000 ("超时毫秒(-1)"), error in (no error)=w362) -> (queue out=w361:refnum<queue>, error out=w360:errorcluster)  [unwired: 1 out]
      }
    }
    n246 = global read "CODCr外部API.vi" "手动模式"() -> (w344:bool)
    n247 = local write "手动模式"(w344) -> ()
    n248 = Get Queue Status(queue=w348, error in (no error)=w347) -> (queue out=w352:refnum<queue>, error out=w351:errorcluster, # elements in queue=w353:i32)  [unwired: 1 in, 5 out]
    n249 = Equal To 0?(x=w353) -> (x = 0?=w350:bool)
    n250 = case shown="真" w350 {
      tunnel: w352 -> [_ w368]
      tunnel: w351 -> [_ w367]
      frame False {
      }
      frame True {
        n251 = Bundle By Name(cluster=cluster{"命令":string} {"命令"=""} ("元素"), "命令"="CODCr读取" ("名称（未命名）")) -> (w370:cluster{"命令":string})
        n252 = Enqueue Element(queue=w368, element=w370, timeout in ms (-1)=1000 ("超时毫秒(-1)"), error in (no error)=w367) -> ()  [unwired: 3 out]
      }
    }
    "主循环次数" <- w354
  }
  n253 = while {
    tunnel: w14 -> [w378]
    tunnel: w13 -> [w377]
    tunnel: [w373] -> _
    stop <- FALSE stop-if-true
    # "CODCr与外部交互"
    n254 = Dequeue Element(queue=w378, error in (no error)=w377) -> (element=w379:T5)  [unwired: 1 in, 3 out]
    n255 = Unbundle By Name(w379) -> ("命令"=w376:string, "测量模式"=w375:T17, "CODCr量程切换"=w374:enum32{"H", "L", "AUTO"})
    n256 = case shown="\"启动命令\"" w376 {
      tunnel: w375 -> [_ w382 _ _]
      tunnel: w374 -> [_ _ _ w412]
      tunnel: [_ w381 w407 w411] -> w373
      frame "假", Default {
      }
      frame "启动命令" {
        n257 = case shown="\"校零\"" w382 {
          tunnel: [u16 4608 ("address") u16 4608 ("address") u16 4608 ("address") u16 4608 ("address") u16 4608 ("address") u16 4608 ("address") u16 4608 ("address") u16 4608 ("address") u16 4608 ("address")] -> w384
          tunnel: [u16 1 ("address") u16 2 ("address") u16 3 ("address") u16 4 ("address") u16 5 ("address") u16 7 ("address") u16 6 ("address") u16 8 ("address") u16 9 ("address")] -> w388
          frame "水样测量" {
          }
          frame "标样核查" {
          }
          frame "零点核查" {
          }
          frame "跨度核查" {
          }
          frame "空白测试" {
          }
          frame "加标回收" {
          }
          frame "平行样" {
          }
          frame "校零" {
          }
          frame "校标" {
          }
        }
        n258 = Insert Into Array(array=u16[] [] ("values"), index=0 ("索引"), new element=w388) -> (w383:u16[])
        n259 = call "CODCrMB_api.vi"("STEP"=enum16{"open", "read", "write", "close"}."write", "values"=w383, "starting address"=w384) -> ("error out"=w381:errorcluster)  [unwired: 6 in, 2 out]
      }
      frame "停止命令" {
        n260 = call "CODCrMB_api.vi"("STEP"=enum16{"open", "read", "write", "close"}."write", "values"=u16[] [12], "starting address"=u16 4608) -> ("error out"=w407:errorcluster)  [unwired: 6 in, 2 out]
      }
      frame "量程切换" {
        n261 = case shown="\"H\"" w412 {
          tunnel: [u16[] [1] ("values") u16[] [0] ("values") _] -> w415
          frame "H" {
          }
          frame "L" {
          }
          frame "AUTO", Default {
          }
        }
        n262 = call "CODCrMB_api.vi"("STEP"=enum16{"open", "read", "write", "close"}."write", "values"=w415, "starting address"=u16 4276) -> ("error out"=w411:errorcluster)  [unwired: 6 in, 2 out]
      }
    }
  }
  n263 = call "Close TimingControl.vi"("error in (no error)"=w2, "TimingControl in"=w3) -> ()  [unwired: 9 in, 1 out]
  n264 = flat-sequence {
    tunnel: w7 -> [_]
    frame #0 {
      n265 = vi-ref "CODCr库.lvlib:关键参数交互.vi"() -> (w425:refnum<vi>)
      n266 = vi-ref "CODCr库.lvlib:CODCr通讯.vi"() -> (w426:refnum<vi>)
      n267 = property class="VI"(reference=w426) -> ("Name"=w427:string)  [unwired: 1 in, 2 out]
      n268 = property class="VI"(reference=w425) -> ("Name"=w424:string)  [unwired: 1 in, 2 out]
      n269 = Open VI Reference(type specifier VI Refnum (for type only)=refnum<vi> refnum, vi path=w427, options=128 ("选项")) -> (vi reference=w429:refnum<vi>, error out=w431:errorcluster)  [unwired: 3 in]
      n270 = Open VI Reference(type specifier VI Refnum (for type only)=refnum<vi> refnum, vi path=w424, options=128 ("选项")) -> (vi reference=w422:refnum<vi>, error out=w420:errorcluster)  [unwired: 3 in]
      n271 = call-by-ref "?"(reference=w429, error in=w431) -> (reference out=w433:refnum<vi>, error out=w432:errorcluster)  [unwired: 12 in]
      n272 = call-by-ref "?"(reference=w422, error in=w420) -> (reference out=w418:refnum<vi>, error out=w419:errorcluster)  [unwired: 12 in]
      n273 = Close Reference(reference=w433, error in (no error)=w432) -> ()  [unwired: 1 out]
      n274 = Close Reference(reference=w418, error in (no error)=w419) -> ()  [unwired: 1 out]
    }
  }
  n275 = while {
    tunnel: [w440] -> _
    shift-right: [w438] -> _
    shift-left: w9 -> [w437]
    tunnel: w8 -> [w434]
    stop <- FALSE stop-if-true
    n276 = Read from Text File(file (use dialog)=w434) -> (text=w438:string, error out=w435:errorcluster)  [unwired: 3 in, 2 out]
    n277 = Not Equal?(x=w438, y=w437) -> (x != y?=w436:bool)
    n278 = Wait (ms)(milliseconds to wait=u32 1000 ("等待时间（毫秒）")) -> ()  [unwired: 1 out]
    n279 = case shown="真" w436 {
      tunnel: [w442 w449] -> w440
      tunnel: w434 -> [_ w443]
      tunnel: w435 -> [w442 _]
      frame False {
      }
      frame True {
        # "文件发生改变进行更新，远端和本地都更新"
        n280 = call <vilib>:"Open Config Data.vi"("configuration file path"=w443) -> ("error out"=w448:errorcluster, "refnum"=w447:T7)  [unwired: 8 in, 1 out]
        n281 = vi-ref "CODCr库.lvlib:CODcr全局变量.vi"() -> (w444:refnum<vi>)
        n282 = call <userlib>:"Read Panel from INI__ogtk.vi"("error in (no error)"=w448, "VI ref"=w444, "refnum"=w447) -> ("error out"=w446:errorcluster, "refnum out"=w445:T7)  [unwired: 7 in]
        n283 = call <vilib>:"Close Config Data.vi"("error in (no error)"=w446, "refnum"=w445) -> ("error out"=w449:errorcluster)  [unwired: 8 in, 1 out]
      }
    }
  }
  n284 = while "While循环" {
    tunnel: w7 -> [_]
    shift-right: [w455] -> _
    shift-left: 0 -> [w456]
    stop <- FALSE stop-if-true
    # "工作状态为空闲时存数据"
    n285 = global read "CODCr外部API.vi" "CODCr外围API"() -> (w458:T19)
    n286 = Wait (ms)(milliseconds to wait=u32 1000 ("等待时间（毫秒）")) -> ()  [unwired: 1 out]
    n287 = global read "CODcr全局变量.vi" "维护模式"() -> (w450:bool)
    n288 = Unbundle By Name(w458) -> ("运行模式"=w451:enum16{"维护模式", "常规模式", "应急模式", "质控模式"})
    n289 = case shown="\"常规模式\", 默认" w451 {
      tunnel: [测试模式."M" ("数据类型") w466] -> w459
      tunnel: w450 -> [_ w467]
      frame "维护模式" {
      }
      frame "常规模式", Default {
        n290 = Select(t=测试模式."M" ("数据类型"), s=w467, f=测试模式."N" ("数据类型")) -> (s? t:f=w466:T18)
      }
    }
    n291 = global read "CODcr全局变量.vi" "状态告警区"() -> (w457:T3)
    n292 = control-ref of="启动测量模式"() -> (w454:refnum<vi>)
    n293 = Unbundle By Name(w457) -> ("工作状态"=w460:u16)
    n294 = call "CODCr数据插入DATA (子VI).vi"("Enum输入"=w454) -> ("data"=w453:T20)  [unwired: 10 in]
    n295 = case shown="0" w460 {
      tunnel: w459 -> [w473 _]
      tunnel: w456 -> [w471 _]
      tunnel: [w472 _] -> w455
      tunnel: w453 -> [w468 _]
      frame 0 {
        n296 = Less Or Equal?(x=w471, y=60) -> (x <= y?=w469:bool)
        n297 = Increment(x=w471) -> (x+1=w472:i32)
        n298 = case shown="真" w469 {
          tunnel: w473 -> [_ w491]
          tunnel: w468 -> [_ w474]
          frame False {
          }
          frame True {
            n299 = local read "启动测量模式"() -> (w483:T1)
            n300 = Equal?(x=T1."水样测试" ("启动测量模式"), y=w483) -> (x = y?=w482:bool)
            n301 = Equal?(x=T1."标样核查" ("启动测量模式"), y=w483) -> (x = y?=w481:bool)
            n302 = Equal?(x=T1."零点核查" ("启动测量模式"), y=w483) -> (x = y?=w480:bool)
            n303 = Equal?(x=T1."跨度核查" ("启动测量模式"), y=w483) -> (x = y?=w479:bool)
            n304 = Equal?(x=T1."空白测试" ("启动测量模式"), y=w483) -> (x = y?=w478:bool)
            n305 = Equal?(x=T1."平行样测试" ("启动测量模式"), y=w483) -> (x = y?=w477:bool)
            n306 = Equal?(x=T1."加标回收" ("启动测量模式"), y=w483) -> (x = y?=w476:bool)
            n307 = Compound Arithmetic op=OR(w482, w481, w480, w479, w478, w477, w476) -> (w475:bool)
            n308 = case shown="真" w475 {
              tunnel: w483 -> [_ w499]
              tunnel: w491 -> [_ w498]
              tunnel: w474 -> [_ w492]
              frame False {
              }
              frame True {
                n309 = global read "CODcr全局变量.vi" "告警状态"() -> (w496:bool)
                n310 = global read "CODcr全局变量.vi" "故障状态"() -> (w495:bool)
                n311 = Or(x=w496, y=w495) -> (x .or. y?=w494:bool)
                n312 = case shown="真" w494 {
                  tunnel: w492 -> [w502 _]
                  tunnel: [w501 "D" ("table")] -> w493
                  frame False {
                    n313 = Unbundle By Name(w502) -> ("数据标识"=w501:string)
                  }
                  frame True {
                    w503 = FALSE ("告警状态")
                    n314 = global write "CODcr全局变量.vi" "告警状态"(w503) -> ()
                    n315 = global write "CODcr全局变量.vi" "故障状态"(w503) -> ()
                  }
                }
                n316 = Bundle By Name(cluster=w492, "因子编码"=u32 1018, "数据标识"=w493) -> (w500:T20)
                n317 = call "CODCr插入数据.vi"("data"=w500, "测量模式"=w499, "数据类型"=w498) -> ()  [unwired: 12 in, 1 out]
              }
            }
          }
        }
      }
      frame 1, Default {
      }
    }
    n318 = Unbundle By Name(w453) -> ("时间标识"=→"数据时间":timestamp)
  }
